vi "VisionGetDistanceAndAngleToSpeaker.vi"() -> (2 "DesiredAngle":dbl, 3 "Distance":dbl)   [LabVIEW 2023]
doc: "From the current robot position (x, y, and angle) and speaker position (central AprilTag) correspnding to current alliance (x and y), returns distance and desired angle to speaker\n--Inputs--None\n--Outputs:\n --Distance to speaker--meters--Numeric\n --Angle to speaker--degress--Numeric"
uses:
  <vilib>/Rock Robotics/WPI/ThirdParty/JAS_Junk/TrajLib/Translation2d_GetXY.vi
  <vilib>/Rock Robotics/WPI/ThirdParty/JAS_Junk/TrajLib/Rotation2d_CreateXY.vi
  <vilib>/Rock Robotics/WPI/ThirdParty/JAS_Junk/TrajLib/Util_CalcDist.vi
  <vilib>/Rock Robotics/WPI/ThirdParty/JAS_Junk/TrajLib/Rotation2d_GetRadians.vi
  <vilib>/Rock Robotics/WPI/ThirdParty/JAS_Junk/TrajLib/Conv_Radians_Deg.vi
  <vilib>/Rock Robotics/WPI/ThirdParty/JAS_Junk/TrajLib/Rotation2d_CreateAngle.vi
  <vilib>/Rock Robotics/WPI/ThirdParty/JAS_Junk/TrajLib/Trajectory_Library.lvlib
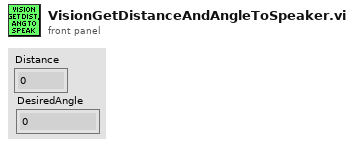
[diagram p1: front panel]
types:
  T1 = typedef "WPI_DriverStationAllianceInfo.ctl" = enum16{"Red", "Blue", "Invalid"}
  T2 = typedef "Trajectory_Library.lvlib/TRANSLATION2D.ctl" = cluster{"X":dbl, "Y":dbl}
  T3 = typedef "Trajectory_Library.lvlib/POSE2D.ctl" = cluster{"TRANSLATION":T2, "ROTATION":T4}
  T4 = typedef "Trajectory_Library.lvlib/ROTATION2D.ctl" = cluster{"VALUE":dbl, "COS":dbl, "SIN":dbl}
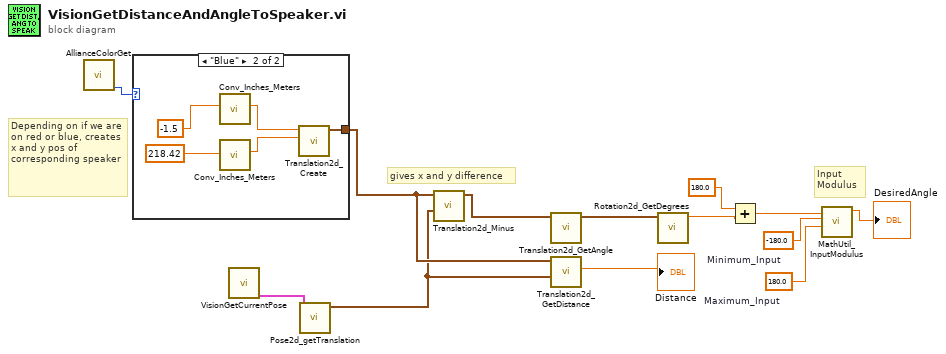
[diagram p0: block diagram]
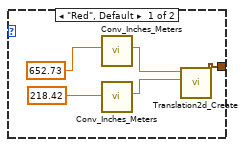
[diagram p2: hidden frame]
diagram:
  w4 = -180.0  # Minimum_Input
  w3 = 180.0  # Maximum_Input
  # "Input\nModulus"
  # "gives x and y difference"
  # "Depending on if we are on red or blue, creates x and y pos of corresponding speaker"
  n1 = call "AllianceColorGet.vi"() -> ("AllianceColor"=w13:T1)  [unwired: 11 in]
  n2 = case shown="\"Blue\"" w13 {
    tunnel: [w14 w19] -> w10
    frame "Red", Default {
      n3 = call <vilib>:"Conv_Inches_Meters.vi"("INCH"=652.73 ("X")) -> ("Meters"=w15:dbl)  [unwired: 10 in]
      n4 = call <vilib>:"Conv_Inches_Meters.vi"("INCH"=218.42 ("Y")) -> ("Meters"=w17:dbl)  [unwired: 10 in]
      n5 = call <vilib>:"Translation2d_Create.vi"("Y"=w17, "X"=w15) -> ("TRANSLATION"=w14:T2)  [unwired: 9 in]
    }
    frame "Blue" {
      n6 = call <vilib>:"Conv_Inches_Meters.vi"("INCH"=-1.5 ("X")) -> ("Meters"=w22:dbl)  [unwired: 10 in]
      n7 = call <vilib>:"Conv_Inches_Meters.vi"("INCH"=218.42 ("Y")) -> ("Meters"=w20:dbl)  [unwired: 10 in]
      n8 = call <vilib>:"Translation2d_Create.vi"("Y"=w20, "X"=w22) -> ("TRANSLATION"=w19:T2)  [unwired: 9 in]
    }
  }
  n9 = call "VisionGetCurrentPose.vi"() -> ("Current Pose"=w12:T3)  [unwired: 9 in]
  n10 = call <vilib>:"Pose2d_getTranslation.vi"("in POSE"=w12) -> ("outTRANSLATION"=w9:T2)  [unwired: 10 in]
  n11 = call <vilib>:"Translation2d_Minus.vi"("other Translation"=w9, "In Translation"=w10) -> ("Out Translation"=w11:T2)  [unwired: 9 in]
  n12 = call <vilib>:"Translation2d_GetAngle.vi"("In Translation"=w11) -> ("Angle_Rotation2d"=w5:T4)  [unwired: 10 in]
  n13 = call <vilib>:"Translation2d_GetDistance.vi"("other Translation"=w9, "In Translation"=w10) -> ("Distance"=→"Distance":dbl)  [unwired: 9 in]
  n14 = call <vilib>:"Rotation2d_GetDegrees.vi"("in ROTATION"=w5) -> ("AngleDegrees"=w7:dbl)  [unwired: 10 in]
  n15 = Add(x=180.0, y=w7) -> (x+y=w2:dbl)
  n16 = call <vilib>:"MathUtil_InputModulus.vi"("Maximum_Input"=w3, "Minimum_Input"=w4, "Input"=w2) -> ("modulus"=→"DesiredAngle":dbl)  [unwired: 8 in]
